vi "GenerateDependencyList.vi"(8 "error in (no error)":errorcluster, 10 "Path to Check":path, 11 "CDependencyInspector in":refnum<class "CDependencyInspection.lvclass">) -> (0 "error out":errorcluster, 1 "Number of Files":i32, 3 "CDependencyInspector out":refnum<class "CDependencyInspection.lvclass">, 4 "Debug string":string)   [LabVIEW 2020, in "DependencyInspection.lvlib" / "CDependencyInspection.lvclass"]
uses:
  CDependencyInspection.lvclass
  CDependencyQueue/CDependencyQueue.lvclass
  CVisitedSet/CVisitedSet.lvclass
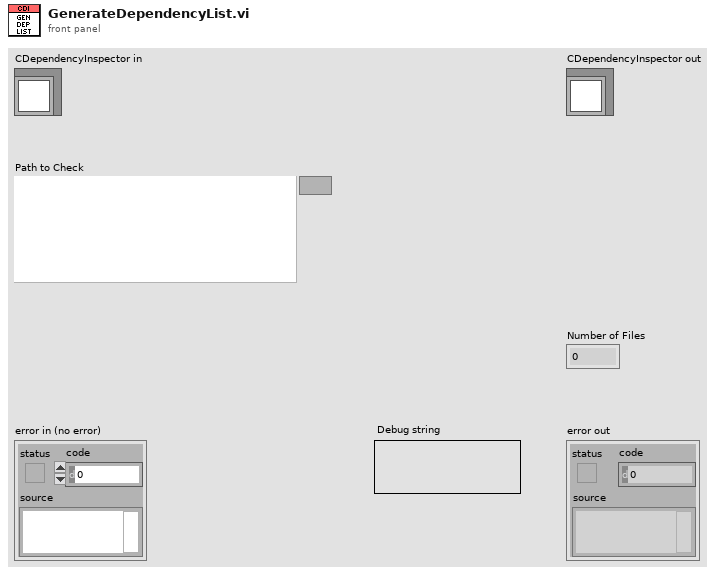
[diagram p1: front panel]
types:
  T1 = typedef "NI_FileType.lvlib/LVFileType.ctl" = enum32{"Invalid file", "Unknown type", "Instrument", "Control", "Polymorphic VI", "Project", "Library", "LVClass", "XControl", "XNode", "Shared library", ".NET assembly", "ActiveX interface", "CIN", "Run-time menu", "Palette menu", "Help file", "LLB", "XNode Edit Dependency", "Class Private Data Control", "Statechart", "MathScript .m file", "Ladder Diagram", "LVLibp", "XNode Build Dependency"}
  T2 = cluster{"path":path, "delimited name":string, "type":T1, "iState":u32, "iStyle":u16, "wStyle":u16, "buttons":u16, "viflags":u32, "viflags2":u32, "links":u32[]}[]
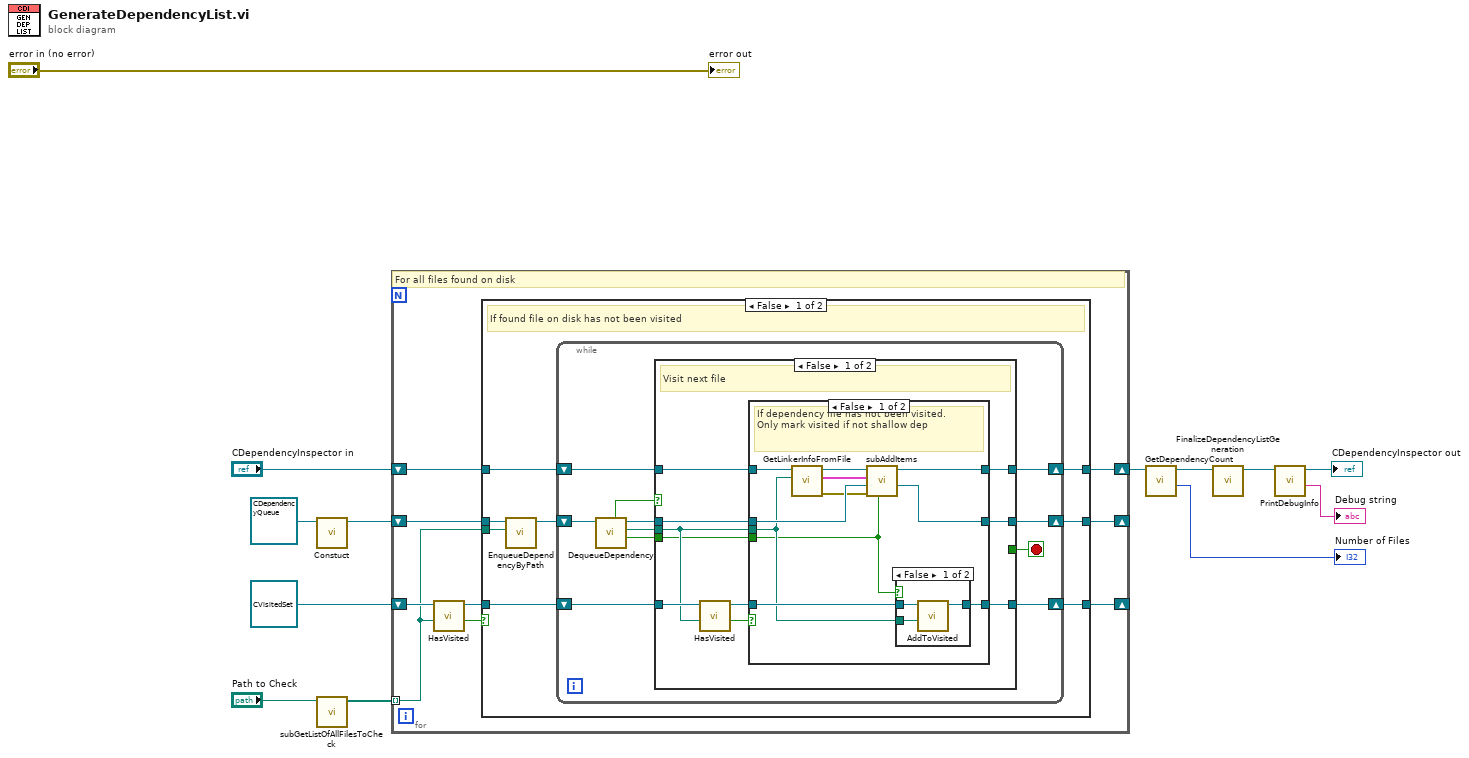
[diagram p0: block diagram]
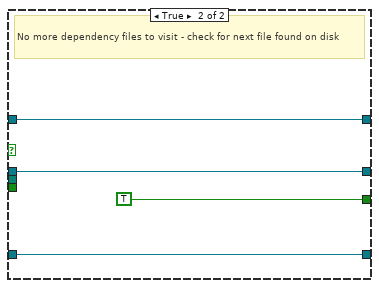
[diagram p4: hidden frame]
diagram:
  n1 = call-dynamic "Constuct.vi"("CDependencyQueue in"=refnum<class "CDependencyQueue.lvclass"> refnum ("DGML_Generator_Helper.lvlib:CDependencyQueue.lvclass")) -> ("CDependencyQueue out"=w10:refnum<class "CDependencyQueue.lvclass">)  [unwired: 9 in, 1 out]
  n2 = call "subGetListOfAllFilesToCheck.vi"("Path to Check"="Path to Check") -> ("All Files in Dir"=w12:path[])  [unwired: 10 in]
  n3 = for {
    tunnel: w12 -> [w14] mode=indexing
    shift-right: [w17] -> w5
    shift-left: "CDependencyInspector in" -> [w22]
    shift-right: [w16] -> _
    shift-left: w10 -> [w21]
    shift-right: [w18] -> _
    shift-left: refnum<class "CVisitedSet.lvclass"> refnum ("DGML_Generator_Helper.lvlib:CVisitedSet.lvclass") -> [w20]
    # "For all files found on disk"
    n4 = call-dynamic "HasVisited.vi"("Path"=w14, "CVisitedSet in"=w20) -> ("found?"=w15:bool, "CVisitedSet out"=w19:refnum<class "CVisitedSet.lvclass">)  [unwired: 7 in, 1 out]
    n5 = case shown="False" w15 {
      tunnel: w22 -> [w30 w76]
      tunnel: w21 -> [w25 w75]
      tunnel: w19 -> [w29 w74]
      tunnel: [w28 w74] -> w18
      tunnel: [w27 w76] -> w17
      tunnel: [w26 w75] -> w16
      tunnel: w14 -> [w23 _]
      frame False {
        # "If found file on disk has not been visited"
        n6 = call-dynamic "EnqueueDependencyByPath.vi"("Path"=w23, "CDependencyQueue in"=w25) -> ("CDependencyQueue out"=w24:refnum<class "CDependencyQueue.lvclass">)  [unwired: 8 in, 1 out]
        n7 = while {
          shift-right: [w38] -> w27
          shift-left: w30 -> [w41]
          shift-right: [w37] -> w26
          shift-left: w24 -> [w36]
          shift-right: [w39] -> w28
          shift-left: w29 -> [w40]
          stop <- w32 stop-if-true
          n8 = call-dynamic "DequeueDependency.vi"("CDependencyQueue in"=w36) -> ("Shallow deps?"=w31:bool, "Path"=w34:path, "CDependencyQueue out"=w35:refnum<class "CDependencyQueue.lvclass">, "timed out?"=w33:bool)  [unwired: 6 in, 1 out]
          n9 = case shown="False" w33 {
            tunnel: w41 -> [w51 w73]
            tunnel: w35 -> [w50 w72]
            tunnel: w40 -> [w49 w71]
            tunnel: [w47 w71] -> w39
            tunnel: [w46 w73] -> w38
            tunnel: [w45 w72] -> w37
            tunnel: w34 -> [w44 _]
            tunnel: [_ TRUE] -> w32
            tunnel: w31 -> [w42 _]
            frame False {
              # "Visit next file"
              n10 = call-dynamic "HasVisited.vi"("Path"=w44, "CVisitedSet in"=w49) -> ("found?"=w43:bool, "CVisitedSet out"=w48:refnum<class "CVisitedSet.lvclass">)  [unwired: 7 in, 1 out]
              n11 = case shown="False" w43 {
                tunnel: w51 -> [w58 w69]
                tunnel: w50 -> [w62 w68]
                tunnel: w48 -> [w61 w67]
                tunnel: [w60 w67] -> w47
                tunnel: [w52 w69] -> w46
                tunnel: [w59 w68] -> w45
                tunnel: w44 -> [w57 _]
                tunnel: w42 -> [w53 _]
                frame False {
                  # "If dependency file has not been visited.\nOnly mark visited if not shallow dep"
                  n12 = call "GetLinkerInfoFromFile.vi"("path in"=w57, "CDependencyInspector in"=w58) -> ("error out"=w55:errorcluster, "Linker.Read Info From File"=w56:T2, "CDependencyInspector out"=w54:refnum<class "CDependencyInspection.lvclass">)  [unwired: 7 in]
                  n13 = call "subAddItems.vi"("Shallow deps?"=w53, "error in (no error)"=w55, "CDependencyQueue in"=w62, "Linker.Read Info From File"=w56, "CDependencyInspector in"=w54) -> ("CDependencyQueue out"=w59:refnum<class "CDependencyQueue.lvclass">, "CDependencyInspector out"=w52:refnum<class "CDependencyInspection.lvclass">)  [unwired: 4 in, 1 out]
                  n14 = case shown="False" w53 {
                    tunnel: w61 -> [w65 w66]
                    tunnel: [w64 w66] -> w60
                    tunnel: w57 -> [w63 _]
                    frame False {
                      n15 = call-dynamic "AddToVisited.vi"("Path"=w63, "CVisitedSet in"=w65) -> ("CVisitedSet out"=w64:refnum<class "CVisitedSet.lvclass">)  [unwired: 8 in, 1 out]
                    }
                    frame True {
                    }
                  }
                }
                frame True {
                  # "Seen this file before"
                }
              }
            }
            frame True {
              # "No more dependency files to visit - check for next file found on disk"
            }
          }
        }
      }
      frame True {
        # "Seen this file before"
      }
    }
  }
  n16 = call-dynamic "GetDependencyCount.vi"("CDependencyInspector in"=w5) -> ("Count"=→"Number of Files":i32, "CDependencyInspector out"=w3:refnum<class "CDependencyInspection.lvclass">)  [unwired: 8 in, 1 out]
  n17 = call-dynamic "FinalizeDependencyListGeneration.vi"("CDependencyInspector in"=w3) -> ("CDependencyInspector out"=w2:refnum<class "CDependencyInspection.lvclass">)  [unwired: 9 in, 1 out]
  n18 = call-dynamic "PrintDebugInfo.vi"("CDependencyInspector in"=w2) -> ("Debug string"=→"Debug string":string, "CDependencyInspector out"=→"CDependencyInspector out":refnum<class "CDependencyInspection.lvclass">)  [unwired: 8 in, 1 out]
  "error out" <- "error in (no error)"
